vi "Write Plot Area Size.vi"(8 "error in (no error)":errorcluster, 10 "PlotAreaSize":T1, 11 "GraphChart.lvclass in":refnum<class "GraphChart.lvclass">) -> (0 "error out":errorcluster, 3 "GraphChart.lvclass out":refnum<class "GraphChart.lvclass">)   [LabVIEW 2015, in "GraphChart.lvclass"]
uses:
  GraphChart.lvclass
  <vilib>/Utility/miscctls.llb/LVBoundsTypeDef.ctl
  GraphChart.lvclass/GraphChart.ctl
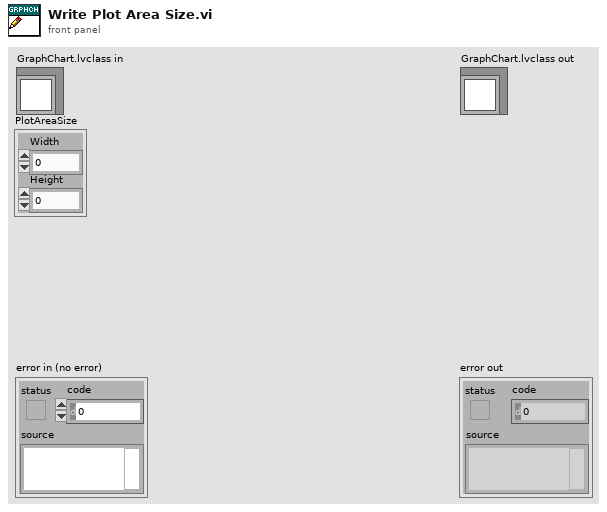
[diagram p1: front panel]
types:
  T1 = typedef "LVBoundsTypeDef.ctl" = cluster{"Width":u32, "Height":u32}
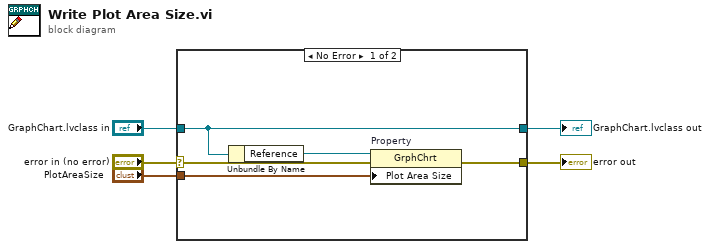
[diagram p0: block diagram]
diagram:
  n1 = case shown="No Error" "error in (no error)" {
    selector: "error in (no error)" -> [w6 w12]
    tunnel: [w10 w12] -> w4
    tunnel: [w8 w11] -> w2
    tunnel: "GraphChart.lvclass in" -> [w8 w11]
    tunnel: "PlotAreaSize" -> [w9 _]
    frame No Error {
      n2 = Unbundle By Name(w8) -> ("Reference"=w7:refnum<vi>)
      n3 = property on="Property" class="GrphChrt"(reference=w7, error in=w6, "Plot Area Size"=w9) -> (error out=w10:errorcluster)  [unwired: 1 out]
    }
    frame Error {
    }
  }
  "error out" <- w4
  "GraphChart.lvclass out" <- w2
